vi "SPC_set_mode.vi"(6 "Modul Type to Simulate":T1 items=["Hardware Modus"=0, "SPC-600 Simulation"=600, "SPC-630 Simulation"=630, "SPC-700  Simulation"=700, "SPC-730  Simulation"=730, "SPC-130  Simulation"=130, "SPC-830  Simulation"=830, "SPC-140  Simulation"=140, "SPC-930  Simulation"=930, "DPC-230  Simulation"=230, "SPC-150  Simulation"=150, "SPC-150 N  Simulation"=151, "SPC-150 NX  Simulation"=152, "SPC-130 EM  Simulation"=131, "SPC-130 EMN  Simulation"=132, "SPC-130 IN Simulation"=135, "SPC-130 INX Simulation"=136, "SPC-130 INXX Simulation"=137, "SPC-160  Simulation"=160, "SPC-160 X  Simulation"=161, "SPC-160 PCIE  Simulation"=162, "SPC-180 Simulation"=180, "SPC-181 Simulation"=181, "SPC-182 Simulation"=182, "SPC-185 Simulation"=185, "SPC-186 Simulation"=186, "SPC-187 Simulation"=187, "DPC-330  Simulation"=330, "DPC-590  Simulation"=590, "TDC-104 Simulation"=104, "TDC-004 Simulation"=4, "TDC-106 Simulation"=106], 7 "Force Use":bool, 8 "Error In":errorcluster, 10 "ModulesToInitalize":i32[](array[numeric]), 11 "DLL Path":path) -> (0 "Error Out":errorcluster, 3 "DLL Path":path)   [LabVIEW 2023]
doc: "Input parameters:\nmode mode of DLL operation\nforce_use force using the module if they are locked ( in use)\n*in_use pointer to the table with information which module must be used\nReturn value: on success - DLL mode, on error <0 (error code)\nThe procedure is used to change the mode of the DLL operation between the hardware mode \nand the simulation mode. It is also used to switch the DLL to the simulation mode if hardware \nerrors occur during the initialisation.\nTable ‘in_use’ should contain entries for all 8 modules:\n0 – means that the module will be unlocked and not used longer\n1 – means that the module will be initialised and locked\nWhen the Hardware Mode is requested for each of 8 possible modules:\n-if ‘in_use’ entry = 1 : the proper module is locked and initialised (if it wasn’t) with the \ninitial parameters set (from ini_file) but only when it was not locked by another \napplication or when ‘force_use’ = 1.\n-if ‘in_use’ entry = 0 : the proper module is unlocked and cannot be used further.\nWhen one of the simulation modes is requested for each of 8 possible modules:\n-if ‘in_use’ entry = 1 : the proper module is initialised (if it wasn’t) with the initial \nparameters set (from ini_file).\n-if ‘in_use’ entry = 0 : the proper module is unlocked and cannot be used further.\nErrors during the module initialisation can cause that the module is excluded from use.\nUse the function SPC_get_init_status and/or SPC_get_module_info to check which modules \nare correctly initialised and can be use further.\nUse the function SPC_get_mode to check which mode is actually set. Possible ‘mode’ values \nare defined in the spcm_def.h file.\n\ninfo@becker-hickl.com"
uses:
  SPC_Controls/ModuleTypes.ctl
panel:
  out "ActualType":i16
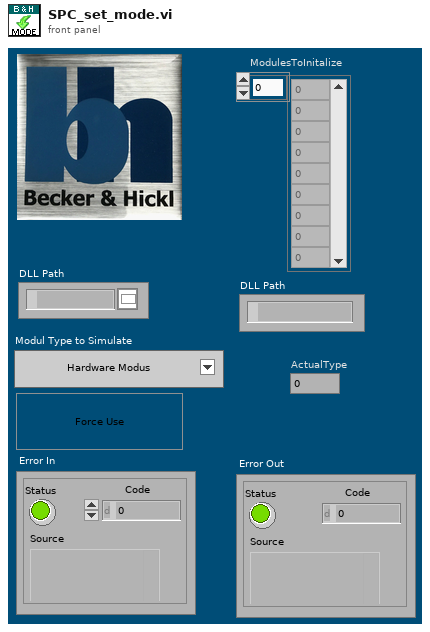
[diagram p1: front panel]
types:
  T1 = typedef "ModuleTypes.ctl" = i16
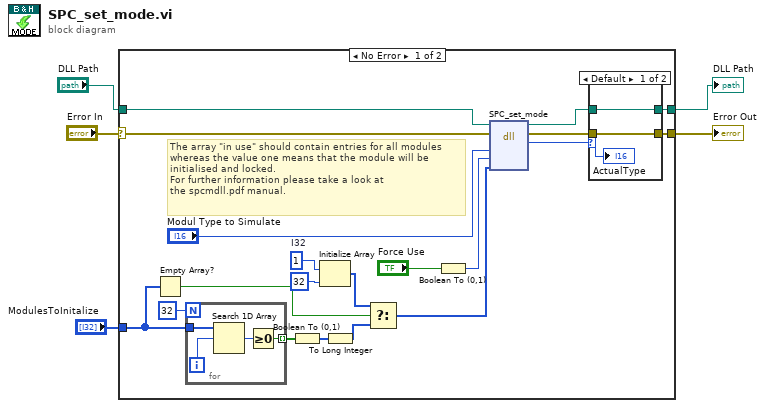
[diagram p0: block diagram]
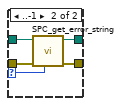
[diagram p2: hidden frame]
diagram:
  n1 = case shown="No Error" "Error In" {
    selector: "Error In" -> [w24 w39]
    tunnel: "DLL Path" -> [w25 w38]
    tunnel: [w20 w39] -> w4
    tunnel: [w19 w38] -> w3
    tunnel: "ModulesToInitalize" -> [w12 _]
    frame No Error {
      w17 = 1  # I32
      # "The array \"in use\" should contain entries for all modules\nwhereas the value one means that the module will be\ninitialised and locked.\nFor further information please take a look at \nthe spcmdll.pdf manual."
      n2 = Empty Array?(array=w12) -> (empty?=w11:bool)
      n3 = for {
        N: 32 -> [_]
        tunnel: w12 -> [w37]
        tunnel: [w34] -> w13 mode=indexing
        i -> [w36]
        n4 = Search 1D Array(1D array=w37, element=w36) -> (index of element=w35:i32)  [unwired: 1 in]
        n5 = Greater Or Equal To 0?(x=w35) -> (x >= 0?=w34:bool)
      }
      n6 = Boolean To (0,1)(Boolean=w13) -> (0, 1=w9:i16[])
      n7 = Initialize Array(w17, 32) -> (w10:i32[])
      n8 = To Long Integer(number=w9) -> (32bit integer=w7:i32[])
      n9 = Select(t=w10, s=w11, f=w7) -> (s? t:f=w8:i32[])
      n10 = Boolean To (0,1)(Boolean="Force Use") -> (0, 1=w23:i16)
      n11 = dll-call lib="D:/spcm/lib/lab_view/lv10.0/spcm32.dll" fn="SPC_set_mode"(path in=w25, error in=w24, "mode"="Modul Type to Simulate", "force_use"=w23, "in_use"=w8) -> (path out=w22:path, error out=w21:errorcluster, "return type"=w6:i16)  [unwired: 4 in]
      n12 = case shown="Default" w6 {
        selector: w6 -> [w26 w29]
        tunnel: w22 -> [w28 w33]
        tunnel: w21 -> [w27 w32]
        tunnel: [w27 w31] -> w20
        tunnel: [w28 w30] -> w19
        frame Default {
          "ActualType" <- w26
        }
        frame ..-1 {
          n13 = call "SPC_get_error_string.vi"("ErrorID"=w29, "Error In"=w32, "DLL Path"=w33) -> ("Error Out"=w31:errorcluster, "DLL Path"=w30:path)  [unwired: 6 in, 1 out]
        }
      }
    }
    frame Error {
    }
  }
  "Error Out" <- w4
  "DLL Path" <- w3
